vi "LoadConfigFile.vi"(8 "error in (no error)":errorcluster, 11 "MatlabExperiment in":refnum<class "MatlabExperiment.lvclass">) -> (0 "error out":errorcluster, 3 "MatlabExperiment out":refnum<class "MatlabExperiment.lvclass">)   [LabVIEW 2014, in "AcquisitionCoreObjects.lvlib" / "MatlabExperiment.lvclass"]
uses:
  MatlabExperiment.lvclass
  Core SubVIs/Controls/TYPE - Configure Test Method.ctl
  <vilib>/Utility/config.llb/Read Key (Path).vi
  Core SubVIs/Core SubVIs.lvlib
  <vilib>/Utility/config.llb/NI_LVConfig.lvlib
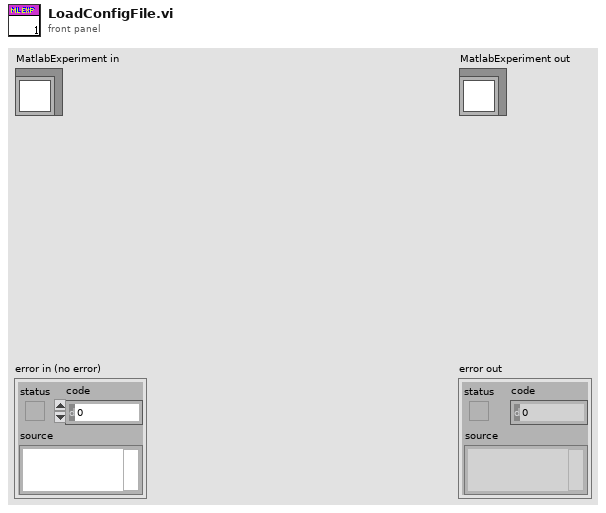
[diagram p1: front panel]
types:
  T1 = typedef "Core SubVIs.lvlib/TYPE - Configure Test Method.ctl" = enum16{"Read Configuration", "Load Configuration from File", "Load from default file", "Configuration Dialog"}
  T2 = typedef "NI_LVConfig.lvlib/Config Data RefNum.ctl" = refnum<k1>
  T3 = cluster{"Name":string, "Type":string, "value":string}[]
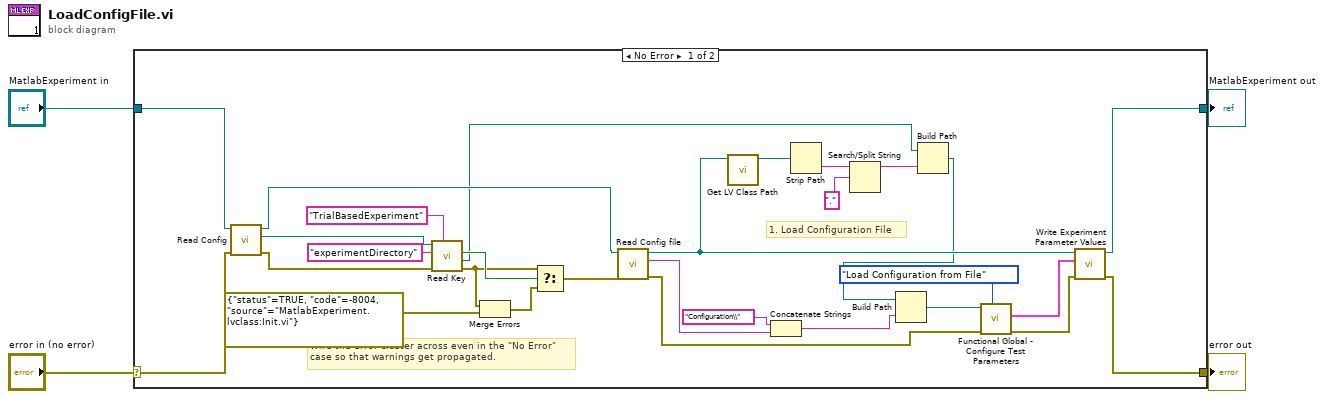
[diagram p0: block diagram]
diagram:
  n1 = case shown="No Error" "error in (no error)" {
    selector: "error in (no error)" -> [w8 w35]
    tunnel: [w7 w35] -> w3
    tunnel: [w5 w34] -> w1
    tunnel: "MatlabExperiment in" -> [w6 w34]
    frame No Error {
      # "1. Load Configuration File"
      # "Wire the error cluster across even in the \"No Error\"\ncase so that warnings get propagated."
      n2 = call-dynamic "Read Config.vi"("error in (no error)"=w8, "AcquistionObject in"=w6) -> ("error out"=w15:errorcluster, "config data"=w24:T2, "AcquistionObject out"=w14:refnum<class "MatlabExperiment.lvclass">)  [unwired: 7 in]
      n3 = call-poly <vilib>:"Read Key.vi"("section"="TrialBasedExperiment", "error in (no error)"=w15, "key"="experimentDirectory", "refnum"=w24) -> ("error out"=w10:errorcluster, "value"=w12:path, "found?"=w21:bool)  [unwired: 4 in, 1 out]
      n4 = Merge Errors(w10, errorcluster {"status"=TRUE, "code"=-8004, "source"="MatlabExperiment.lvclass:Init.vi"} ("f")) -> (w9:errorcluster)
      n5 = Select(t=w10, s=w21, f=w9) -> (s? t:f=w13:errorcluster)
      n6 = call-dynamic "Read Config file.vi"("error in (no error)"=w13, "TrialBasedExperiment in"=w14) -> ("error out"=w28:errorcluster, "Config file"=w29:string, "TrialBasedExperiment out"=w25:refnum<class "MatlabExperiment.lvclass">)  [unwired: 7 in]
      n7 = call <vilib>:"Get LV Class Path.vi"("object"=w25) -> ("class path"=w19:path)  [unwired: 9 in, 1 out]
      n8 = Concatenate Strings("Configuration\\" ("name or relative path"), w29) -> (w30:string)
      n9 = Strip Path(path=w19) -> (name=w20:string)  [unwired: 1 out]
      n10 = Search/Split String(string=w20, search string/char (-)=".") -> (substring before match=w17:string)  [unwired: 1 in, 2 out]
      n11 = Build Path(base path=w12, name or relative path=w17) -> (appended path=w16:path)
      n12 = Build Path(base path=w16, name or relative path=w30) -> (appended path=w32:path)
      n13 = call "Functional Global - Configure Test Parameters.vi"("Configure Test Method"=TYPE_-_Configure_Test_Method."Load Configuration from File", "error in (no error)"=w28, "Paramater Definition File Path"=w32) -> ("error out"=w26:errorcluster, "Experiment Parameter Values"=w27:T3)  [unwired: 7 out]
      n14 = call-dynamic "Write Experiment Parameter Values.vi"("error in (no error)"=w26, "Experiment Parameter Values"=w27, "TrialBasedExperiment in"=w25) -> ("error out"=w7:errorcluster, "TrialBasedExperiment out"=w5:refnum<class "MatlabExperiment.lvclass">)  [unwired: 7 in]
    }
    frame Error {
    }
  }
  "error out" <- w3
  "MatlabExperiment out" <- w1
